vi "Status Register.vi"(8 "error in (no error)":errorcluster, 9 "Register Bit(0)":dbl min=0.0 max=255.0 step=1.0, 10 "Status Register(0:Quest Event Enable Register)":u16(ring) items=["Quest Event Enable Register", "Quest Event Enable Register?", "Quest Event Register?", "Quest Condition register?", "Operation Event Enable Register", "Operation Event Enable Register?", "Operation Event Register?", "Operation Condition Register?"], 11 "VISA resource name":refnum<visa-resource-name>) -> (0 "error out":errorcluster, 2 "Status Register Response":string, 3 "VISA resource name out":refnum<visa-resource-name>)   [LabVIEW 2021, in "Keithley 2200 Series.lvlib"]
doc: "Sends query to the power supply and obtains the response from the instrument and sets particular bit of the specified register to 1."
uses:
  <instrlib>/Keithley 2200 Series/Keithley 2200 Series.lvlib
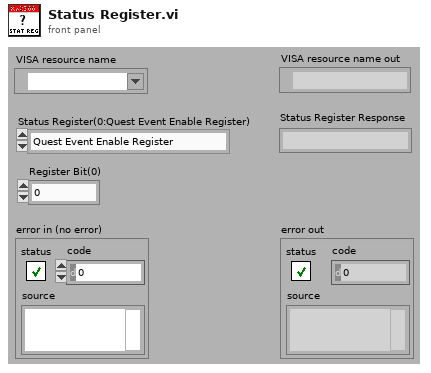
[diagram p1: front panel]
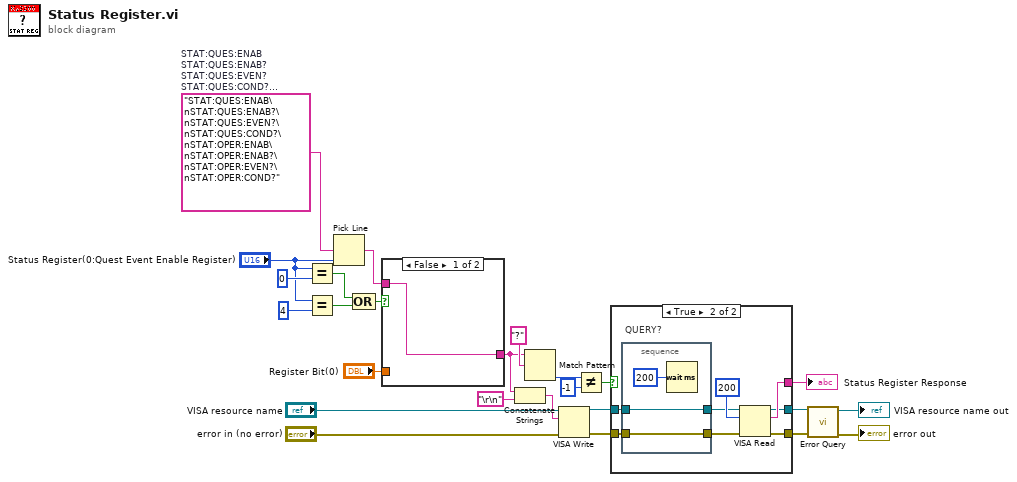
[diagram p0: block diagram]
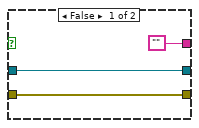
[diagram p2: hidden frame]
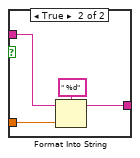
[diagram p3: hidden frame]
diagram:
  w23 = "STAT:QUES:ENAB\nSTAT:QUES:ENAB?\nSTAT:QUES:EVEN?\nSTAT:QUES:COND?\nSTAT:OPER:ENAB\nSTAT:OPER:ENAB?\nSTAT:OPER:EVEN?\nSTAT:OPER:COND?"  # STAT:QUES:ENAB STAT:QUES:ENAB? STAT:QUES:EVEN? STAT:QUES:COND? STAT:OPER:ENAB STAT:OPER:ENAB? STAT:OPER:EVEN? STAT:OPER:COND?
  n1 = Equal?(x="Status Register(0:Quest Event Enable Register)", y=u16 0) -> (x = y?=w22:bool)
  n2 = Equal?(x="Status Register(0:Quest Event Enable Register)", y=u16 4) -> (x = y?=w21:bool)
  n3 = Pick Line(multi-line string=w23, line index="Status Register(0:Quest Event Enable Register)") -> (output string=w17:string)  [unwired: 1 out]
  n4 = Compound Arithmetic op=OR(w22, w21) -> (w16:bool)
  n5 = case shown="False" w16 {
    tunnel: [w26 w29] -> w7
    tunnel: "Register Bit(0)" -> [_ w28]
    tunnel: w17 -> [w26 w27]
    frame False {
    }
    frame True {
      n6 = Format Into String(format string=" %d", initial string=w27, w28) -> (resulting string=w29:string)  [unwired: 1 in, 1 out]
    }
  }
  n7 = Concatenate Strings(w7, "\r\n" ("End of Line Constant")) -> (w12:string)
  n8 = Match Pattern(string=w7, regular expression="?") -> (offset past match=w9:i32)  [unwired: 4 out]
  n9 = VISA Write(VISA resource name="VISA resource name", write buffer=w12, error in (no error)="error in (no error)") -> (VISA resource name out=w15:refnum<visa-resource-name>, error out=w14:errorcluster)  [unwired: 1 out]
  n10 = Not Equal?(x=w9, y=-1) -> (x != y?=w6:bool)
  n11 = case shown="True" w6 {
    tunnel: w15 -> [w32 w40]
    tunnel: w14 -> [w31 w39]
    tunnel: ["" ("read buffer") w36] -> w5
    tunnel: [w32 w35] -> w4
    tunnel: [w31 w34] -> w3
    frame False {
    }
    frame True {
      # "QUERY?"
      n12 = stacked-sequence {
        tunnel: w40 -> [w43]
        tunnel: w39 -> [w42]
        tunnel: [w43] -> w38
        tunnel: [w42] -> w37
        frame #0 {
          n13 = Wait (ms)(milliseconds to wait=u32 200) -> ()  [unwired: 1 out]
        }
      }
      n14 = VISA Read(VISA resource name=w38, byte count=u32 200, error in (no error)=w37) -> (VISA resource name out=w35:refnum<visa-resource-name>, read buffer=w36:string, error out=w34:errorcluster)  [unwired: 1 out]
    }
  }
  "Status Register Response" <- w5
  n15 = call <instrlib>:"Error Query.vi"("error in (no error)"=w3, "VISA resource name"=w4) -> ("error out"=→"error out":errorcluster, "VISA resource name out"=→"VISA resource name out":refnum<visa-resource-name>)  [unwired: 8 out]
